vi "Send Blend Wrapper.vi"(7 "Include Source EnQr (T)":bool=TRUE, 8 "error in (no error)":errorcluster, 9 "Sample to Blend":refnum<class "Sample.lvclass">, 10 "Send to":refnum<class "Message Enqueuer.lvclass">[](array[class]), 11 "CO2 Actor in":refnum<class "CO2 Actor.lvclass">) -> (0 "error out":errorcluster, 3 "CO2 Actor out":refnum<class "CO2 Actor.lvclass">)   [LabVIEW 2015, in "cRIO-Carbondioxide.lvlib" / "CO2-Actor.lvlib" / "CO2 Actor.lvclass"]
uses:
  CO2 Actor.lvclass
  subs/Sample/Sample.lvclass
  <vilib>/ActorFramework/Message Enqueuer/Message Enqueuer.lvclass
  <vilib>/ActorFramework/Actor/Actor.lvclass/Actor.ctl
  <vilib>/ActorFramework/Message Enqueuer/Message Enqueuer.lvclass/Message Enqueuer.ctl
  CO2 Actor.lvclass/CO2 Actor.ctl
  <vilib>/ActorFramework/Message Enqueuer/Message Priority.ctl
  CO2 Actor Messages/Blend Msg/Blend Msg.lvclass/Blend Msg.ctl
  <vilib>/ActorFramework/Message Enqueuer/Enqueue.vi
  <vilib>/ActorFramework/Actor/Read Self Enqueuer.vi
  <vilib>/ActorFramework/Message Enqueuer/Init from Existing Queue.vi
  <vilib>/ActorFramework/Message Priority Queue/Priority Enqueue.vi
  CO2 Actor Messages/Blend Msg/Blend Msg.lvclass
  <vilib>/ActorFramework/Actor/Actor.lvclass
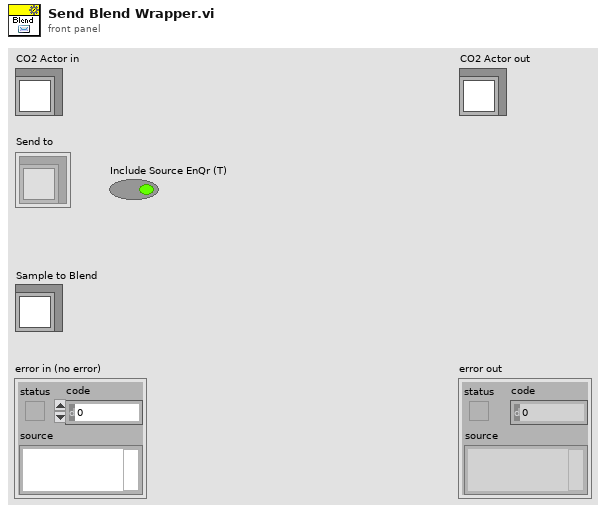
[diagram p1: front panel]
types:
  T1 = typedef "Actor Framework.lvlib/Message Enqueuer.lvclass/Message Priority.ctl" = enum16{"Low", "Normal", "High"}
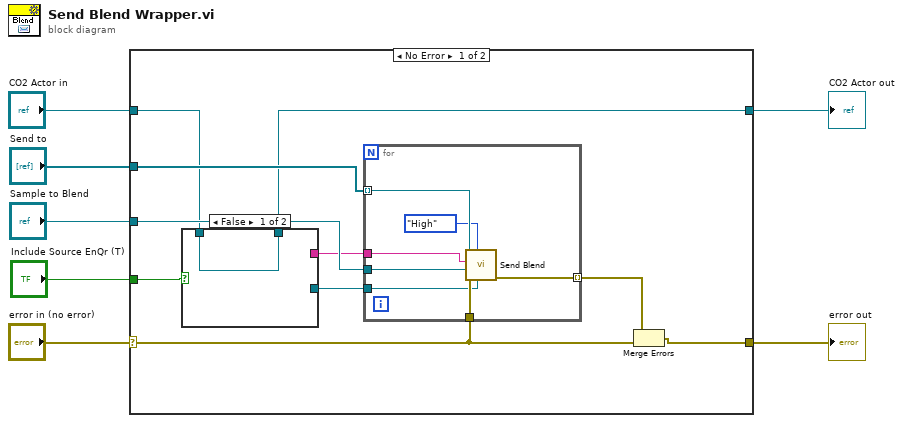
[diagram p0: block diagram]
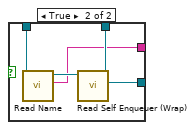
[diagram p2: hidden frame]
diagram:
  n1 = case shown="No Error" "error in (no error)" {
    selector: "error in (no error)" -> [w16 w32]
    tunnel: [w17 w32] -> w6
    tunnel: "CO2 Actor in" -> [w9 w31]
    tunnel: [w10 w31] -> w4
    tunnel: "Sample to Blend" -> [w12 _]
    tunnel: "Send to" -> [w13 _]
    tunnel: "Include Source EnQr (T)" -> [w11 _]
    frame No Error {
      n2 = case shown="False" w11 {
        tunnel: [_ w23] -> w14
        tunnel: w9 -> [w18 w21]
        tunnel: [w18 w22] -> w10
        tunnel: [_ w19] -> w8
        frame False {
        }
        frame True {
          n3 = call "Read Name.vi"("CO2 Actor in"=w21) -> ("Name"=w19:string, "CO2 Actor out"=w20:refnum<class "CO2 Actor.lvclass">)  [unwired: 9 in]
          n4 = call "Read Self Enqueuer (Wrap).vi"("CO2 Actor in"=w20) -> ("Actor Framework:Message Enqueuer"=w23:refnum<class "Message Enqueuer.lvclass">, "CO2 Actor out"=w22:refnum<class "CO2 Actor.lvclass">)  [unwired: 9 in]
        }
      }
      n5 = for {
        tunnel: w13 -> [w27] mode=indexing
        tunnel: w16 -> [w30]
        tunnel: [w29] -> w15 mode=indexing
        tunnel: w12 -> [w28]
        tunnel: w14 -> [w26]
        tunnel: w8 -> [w25]
        n6 = call "Send Blend.vi"("Source Enqueuer"=w26, "Message Priority (Normal)"=Message_Priority."High", "error in (no error)"=w30, "Sample to Blend"=w28, "Source Name"=w25, "Message Enqueuer"=w27) -> ("error out"=w29:errorcluster)  [unwired: 4 in, 1 out]
      }
      n7 = Merge Errors(w15, w16) -> (w17:errorcluster)
    }
    frame Error {
    }
  }
  "error out" <- w6
  "CO2 Actor out" <- w4
